vi "Add Command.vi"(6 "Notification?(F)":bool, 8 "error in (no error)":errorcluster, 9 "Type Descriptor":string, 10 "Command Name":string, 11 "DIMActor in":refnum<class "DIMActor.lvclass">) -> (0 "error out":errorcluster, 3 "DIMActor out":refnum<class "DIMActor.lvclass">)   [LabVIEW 2012, in "DIMActor.lvlib" / "DIMActor.lvclass"]
doc: "Plublish a DIM command."
uses:
  DIMActor.lvclass
  DIMActor.lvclass/DIMActor.ctl
  SVN/LV2009/GPL/lib.lib/DimLVEvent/LVDimInterface/LVDimInterface.dis_add_command_notifier.vi
  SVN/LV2009/GPL/lib.lib/DimLVEvent/LVDimInterface/LVDimInterface.dis_add_command_queue.vi
  SVN/LV2009/GPL/lib.lib/DimLVEvent/LVDimInterface/LVDimInterface.lvlib
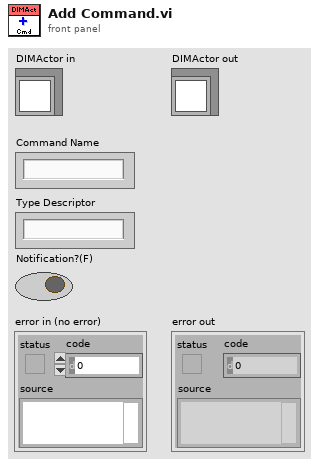
[diagram p1: front panel]
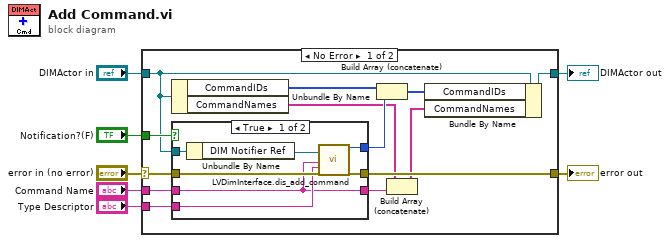
[diagram p0: block diagram]
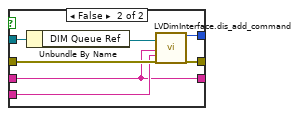
[diagram p2: hidden frame]
diagram:
  n1 = case shown="No Error" "error in (no error)" {
    selector: "error in (no error)" -> [w20 w36]
    tunnel: [w19 w36] -> w6
    tunnel: [w11 w35] -> w4
    tunnel: "DIMActor in" -> [w12 w35]
    tunnel: "Command Name" -> [w18 _]
    tunnel: "Type Descriptor" -> [w17 _]
    tunnel: "Notification?(F)" -> [w13 _]
    frame No Error {
      n2 = Unbundle By Name(w12) -> ("CommandIDs"=w14:i32[], "CommandNames"=w10:string[])
      n3 = case shown="True" w13 {
        tunnel: w20 -> [w27 w34]
        tunnel: [w26 w33] -> w19
        tunnel: w18 -> [w21 w28]
        tunnel: w17 -> [w25 w32]
        tunnel: [w24 w31] -> w16
        tunnel: w12 -> [w23 w30]
        tunnel: [w21 w28] -> w9
        frame True {
          n4 = Unbundle By Name(w23) -> ("DIM Notifier Ref"=w22:refnum<notifier>)
          n5 = call-poly "LVDimInterface.dis_add_command.vi"("notifier"=w22, "commandName"=w21, "typeDescriptor"=w25, "error in (no error)"=w27) -> ("commandID"=w24:i32, "error out"=w26:errorcluster)  [unwired: 14 in]
        }
        frame False {
          n6 = Unbundle By Name(w30) -> ("DIM Queue Ref"=w29:refnum<queue>)
          n7 = call-poly "LVDimInterface.dis_add_command.vi"("queueRef"=w29, "commandName"=w28, "typeDescriptor"=w32, "error in (no error)"=w34) -> ("commandID"=w31:i32, "error out"=w33:errorcluster)  [unwired: 14 in]
        }
      }
      n8 = Build Array (concatenate)(w14, w16) -> (w15:i32[])
      n9 = Build Array (concatenate)(w10, w9) -> (w8:string[])
      n10 = Bundle By Name(cluster=w12, "CommandIDs"=w15, "CommandNames"=w8) -> (w11:refnum<class "DIMActor.lvclass">)
    }
    frame Error {
    }
  }
  "error out" <- w6
  "DIMActor out" <- w4
